vi "process.vi"(4 "error in":errorcluster, 6 "vars runtime":T1[](array[typedef])=[{"t wait"=5000, "t stim"=0, "t square"=0, "t rew"=0, "t onset"=0, "n stim"=0, "n hit"=0, "n miss"=0, "n catch"=0, "n reject"=0, "n false alarm"=0, "stim amp"=0.0, "stim idx"=0, "next temp"=0.0, "catch"=FALSE, "stimulus"=FALSE, "reward given"=FALSE, "lick"=FALSE, "next reward"=FALSE, "backlight"=FALSE, "square"=FALSE, "first run?"=TRUE, "run square?"=FALSE, "timeout"=FALSE, "free reward"=FALSE, "d stim"=0, "d square"=0, "n rew"=0}, {"t wait"=5000, "t stim"=0, "t square"=0, "t rew"=0, "t onset"=0, "n stim"=0, "n hit"=0, "n miss"=0, "n catch"=0, "n reject"=0, "n false alarm"=0, "stim amp"=0.0, "stim idx"=0, "next temp"=0.0, "catch"=FALSE, "stimulus"=FALSE, "reward given"=FALSE, "lick"=FALSE, "next reward"=FALSE, "backlight"=FALSE, "square"=FALSE, "first run?"=TRUE, "run square?"=FALSE, "timeout"=FALSE, "free reward"=FALSE, "d stim"=0, "d square"=0, "n rew"=0}, {"t wait"=5000, "t stim"=0, "t square"=0, "t rew"=0, "t onset"=0, "n stim"=0, "n hit"=0, "n miss"=0, "n catch"=0, "n reject"=0, "n false alarm"=0, "stim amp"=0.0, "stim idx"=0, "next temp"=0.0, "catch"=FALSE, "stimulus"=FALSE, "reward given"=FALSE, "lick"=FALSE, "next reward"=FALSE, "backlight"=FALSE, "square"=FALSE, "first run?"=TRUE, "run square?"=FALSE, "timeout"=FALSE, "free reward"=FALSE, "d stim"=0, "d square"=0, "n rew"=0}, {"t wait"=5000, "t stim"=0, "t square"=0, "t rew"=0, "t onset"=0, "n stim"=0, "n hit"=0, "n miss"=0, "n catch"=0, "n reject"=0, "n false alarm"=0, "stim amp"=0.0, "stim idx"=0, "next temp"=0.0, "catch"=FALSE, "stimulus"=FALSE, "reward given"=FALSE, "lick"=FALSE, "next reward"=FALSE, "backlight"=FALSE, "square"=FALSE, "first run?"=TRUE, "run square?"=FALSE, "timeout"=FALSE, "free reward"=FALSE, "d stim"=0, "d square"=0, "n rew"=0}], 7 "vars general":T2[](array[typedef])=[{"base directory"=path "C:/Users/training/Desktop/Data", "data directory"=path "C:/Users/training/Desktop/Data/animal001/session064", "active"=FALSE, "running"=FALSE, "pairing"=FALSE, "clean tubes"=FALSE, "animal ID"=1, "session ID"=64, "base temp"=32.0, "d wait min"=500, "d wait max"=1000, "d timeout"=5000, "d reward"=100, "n reward"=1, "idx stim"=0, "timeout win"=5000, "lick win"=[0, 100], "stim type"=[enum."pulse", enum."sine", enum."square"], "stim dur"=[500, 700, 600], "stim amp"=[10.0, 10.0, 10.0], "stim freq"=[50, 50, 50], "stim ramp"=[50, 1, 1], "stim catch"=[0, 0, 1], "square dur"=[50, 20, 10], "square delay"=[50, 20, 10], "square freq"=[50, 50, 50], "square dc"=[50, 20, 10], "stim shape"=array3x700[2100 elements], "square shape"=[[TRUE, TRUE, TRUE, TRUE, TRUE, TRUE, TRUE, TRUE, TRUE, TRUE, FALSE, FALSE, FALSE, FALSE, FALSE, FALSE, FALSE, FALSE, FALSE, FALSE, TRUE, TRUE, TRUE, TRUE, TRUE, TRUE, TRUE, TRUE, TRUE, TRUE, FALSE, FALSE, FALSE, FALSE, FALSE, FALSE, FALSE, FALSE, FALSE, FALSE, TRUE, TRUE, TRUE, TRUE, TRUE, TRUE, TRUE, TRUE, TRUE, TRUE], [TRUE, TRUE, TRUE, TRUE, FALSE, FALSE, FALSE, FALSE, FALSE, FALSE, FALSE, FALSE, FALSE, FALSE, FALSE, FALSE, FALSE, FALSE, FALSE, FALSE, FALSE, FALSE, FALSE, FALSE, FALSE, FALSE, FALSE, FALSE, FALSE, FALSE, FALSE, FALSE, FALSE, FALSE, FALSE, FALSE, FALSE, FALSE, FALSE, FALSE, FALSE, FALSE, FALSE, FALSE, FALSE, FALSE, FALSE, FALSE, FALSE, FALSE], [TRUE, TRUE, FALSE, FALSE, FALSE, FALSE, FALSE, FALSE, FALSE, FALSE, FALSE, FALSE, FALSE, FALSE, FALSE, FALSE, FALSE, FALSE, FALSE, FALSE, FALSE, FALSE, FALSE, FALSE, FALSE, FALSE, FALSE, FALSE, FALSE, FALSE, FALSE, FALSE, FALSE, FALSE, FALSE, FALSE, FALSE, FALSE, FALSE, FALSE, FALSE, FALSE, FALSE, FALSE, FALSE, FALSE, FALSE, FALSE, FALSE, FALSE]]}, {"base directory"=path "C:/Users/training/Desktop/Data", "data directory"=path "C:/Users/training/Desktop/Data/animal002/session122", "active"=FALSE, "running"=FALSE, "pairing"=FALSE, "clean tubes"=FALSE, "animal ID"=2, "session ID"=122, "base temp"=32.0, "d wait min"=500, "d wait max"=1000, "d timeout"=5000, "d reward"=100, "n reward"=1, "idx stim"=0, "timeout win"=5000, "lick win"=[0, 100], "stim type"=[enum."pulse", enum."sine", enum."square"], "stim dur"=[500, 700, 600], "stim amp"=[10.0, 10.0, 10.0], "stim freq"=[50, 50, 50], "stim ramp"=[50, 1, 1], "stim catch"=[0, 0, 1], "square dur"=[50, 20, 10], "square delay"=[50, 20, 10], "square freq"=[50, 50, 50], "square dc"=[50, 20, 10], "stim shape"=array3x700[2100 elements], "square shape"=[[TRUE, TRUE, TRUE, TRUE, TRUE, TRUE, TRUE, TRUE, TRUE, TRUE, FALSE, FALSE, FALSE, FALSE, FALSE, FALSE, FALSE, FALSE, FALSE, FALSE, TRUE, TRUE, TRUE, TRUE, TRUE, TRUE, TRUE, TRUE, TRUE, TRUE, FALSE, FALSE, FALSE, FALSE, FALSE, FALSE, FALSE, FALSE, FALSE, FALSE, TRUE, TRUE, TRUE, TRUE, TRUE, TRUE, TRUE, TRUE, TRUE, TRUE], [TRUE, TRUE, TRUE, TRUE, FALSE, FALSE, FALSE, FALSE, FALSE, FALSE, FALSE, FALSE, FALSE, FALSE, FALSE, FALSE, FALSE, FALSE, FALSE, FALSE, FALSE, FALSE, FALSE, FALSE, FALSE, FALSE, FALSE, FALSE, FALSE, FALSE, FALSE, FALSE, FALSE, FALSE, FALSE, FALSE, FALSE, FALSE, FALSE, FALSE, FALSE, FALSE, FALSE, FALSE, FALSE, FALSE, FALSE, FALSE, FALSE, FALSE], [TRUE, TRUE, FALSE, FALSE, FALSE, FALSE, FALSE, FALSE, FALSE, FALSE, FALSE, FALSE, FALSE, FALSE, FALSE, FALSE, FALSE, FALSE, FALSE, FALSE, FALSE, FALSE, FALSE, FALSE, FALSE, FALSE, FALSE, FALSE, FALSE, FALSE, FALSE, FALSE, FALSE, FALSE, FALSE, FALSE, FALSE, FALSE, FALSE, FALSE, FALSE, FALSE, FALSE, FALSE, FALSE, FALSE, FALSE, FALSE, FALSE, FALSE]]}, {"base directory"=path "C:/Users/training/Desktop/Data", "data directory"=path "C:/Users/training/Desktop/Data/animal003/session155", "active"=FALSE, "running"=FALSE, "pairing"=FALSE, "clean tubes"=FALSE, "animal ID"=3, "session ID"=155, "base temp"=32.0, "d wait min"=500, "d wait max"=1000, "d timeout"=5000, "d reward"=100, "n reward"=1, "idx stim"=0, "timeout win"=5000, "lick win"=[0, 100], "stim type"=[enum."pulse", enum."sine", enum."square"], "stim dur"=[500, 700, 600], "stim amp"=[10.0, 10.0, 10.0], "stim freq"=[50, 50, 50], "stim ramp"=[50, 1, 1], "stim catch"=[0, 0, 1], "square dur"=[50, 20, 10], "square delay"=[50, 20, 10], "square freq"=[50, 50, 50], "square dc"=[50, 20, 10], "stim shape"=array3x700[2100 elements], "square shape"=[[TRUE, TRUE, TRUE, TRUE, TRUE, TRUE, TRUE, TRUE, TRUE, TRUE, FALSE, FALSE, FALSE, FALSE, FALSE, FALSE, FALSE, FALSE, FALSE, FALSE, TRUE, TRUE, TRUE, TRUE, TRUE, TRUE, TRUE, TRUE, TRUE, TRUE, FALSE, FALSE, FALSE, FALSE, FALSE, FALSE, FALSE, FALSE, FALSE, FALSE, TRUE, TRUE, TRUE, TRUE, TRUE, TRUE, TRUE, TRUE, TRUE, TRUE], [TRUE, TRUE, TRUE, TRUE, FALSE, FALSE, FALSE, FALSE, FALSE, FALSE, FALSE, FALSE, FALSE, FALSE, FALSE, FALSE, FALSE, FALSE, FALSE, FALSE, FALSE, FALSE, FALSE, FALSE, FALSE, FALSE, FALSE, FALSE, FALSE, FALSE, FALSE, FALSE, FALSE, FALSE, FALSE, FALSE, FALSE, FALSE, FALSE, FALSE, FALSE, FALSE, FALSE, FALSE, FALSE, FALSE, FALSE, FALSE, FALSE, FALSE], [TRUE, TRUE, FALSE, FALSE, FALSE, FALSE, FALSE, FALSE, FALSE, FALSE, FALSE, FALSE, FALSE, FALSE, FALSE, FALSE, FALSE, FALSE, FALSE, FALSE, FALSE, FALSE, FALSE, FALSE, FALSE, FALSE, FALSE, FALSE, FALSE, FALSE, FALSE, FALSE, FALSE, FALSE, FALSE, FALSE, FALSE, FALSE, FALSE, FALSE, FALSE, FALSE, FALSE, FALSE, FALSE, FALSE, FALSE, FALSE, FALSE, FALSE]]}, {"base directory"=path "C:/Users/training/Desktop/Data", "data directory"=path "C:/Users/training/Desktop/Data/animal004/session061", "active"=FALSE, "running"=FALSE, "pairing"=FALSE, "clean tubes"=FALSE, "animal ID"=4, "session ID"=61, "base temp"=32.0, "d wait min"=500, "d wait max"=1000, "d timeout"=5000, "d reward"=100, "n reward"=1, "idx stim"=0, "timeout win"=5000, "lick win"=[0, 100], "stim type"=[enum."pulse", enum."sine", enum."square"], "stim dur"=[500, 700, 595], "stim amp"=[10.0, 10.0, 10.0], "stim freq"=[50, 50, 50], "stim ramp"=[50, 1, 1], "stim catch"=[0, 0, 1], "square dur"=[50, 20, 10], "square delay"=[50, 20, 10], "square freq"=[50, 50, 50], "square dc"=[50, 20, 10], "stim shape"=array3x700[2100 elements], "square shape"=[[TRUE, TRUE, TRUE, TRUE, TRUE, TRUE, TRUE, TRUE, TRUE, TRUE, FALSE, FALSE, FALSE, FALSE, FALSE, FALSE, FALSE, FALSE, FALSE, FALSE, TRUE, TRUE, TRUE, TRUE, TRUE, TRUE, TRUE, TRUE, TRUE, TRUE, FALSE, FALSE, FALSE, FALSE, FALSE, FALSE, FALSE, FALSE, FALSE, FALSE, TRUE, TRUE, TRUE, TRUE, TRUE, TRUE, TRUE, TRUE, TRUE, TRUE], [TRUE, TRUE, TRUE, TRUE, FALSE, FALSE, FALSE, FALSE, FALSE, FALSE, FALSE, FALSE, FALSE, FALSE, FALSE, FALSE, FALSE, FALSE, FALSE, FALSE, FALSE, FALSE, FALSE, FALSE, FALSE, FALSE, FALSE, FALSE, FALSE, FALSE, FALSE, FALSE, FALSE, FALSE, FALSE, FALSE, FALSE, FALSE, FALSE, FALSE, FALSE, FALSE, FALSE, FALSE, FALSE, FALSE, FALSE, FALSE, FALSE, FALSE], [TRUE, TRUE, FALSE, FALSE, FALSE, FALSE, FALSE, FALSE, FALSE, FALSE, FALSE, FALSE, FALSE, FALSE, FALSE, FALSE, FALSE, FALSE, FALSE, FALSE, FALSE, FALSE, FALSE, FALSE, FALSE, FALSE, FALSE, FALSE, FALSE, FALSE, FALSE, FALSE, FALSE, FALSE, FALSE, FALSE, FALSE, FALSE, FALSE, FALSE, FALSE, FALSE, FALSE, FALSE, FALSE, FALSE, FALSE, FALSE, FALSE, FALSE]]}] {"stim ramp" min=1}) -> (0 "error out":errorcluster, 2 "vars runtime":T1[](array[typedef])=[{"t wait"=5000, "t stim"=0, "t square"=0, "t rew"=0, "t onset"=0, "n stim"=0, "n hit"=0, "n miss"=0, "n catch"=0, "n reject"=0, "n false alarm"=0, "stim amp"=0.0, "stim idx"=0, "next temp"=32.0, "catch"=FALSE, "stimulus"=FALSE, "reward given"=FALSE, "lick"=FALSE, "next reward"=FALSE, "backlight"=FALSE, "square"=FALSE, "first run?"=TRUE, "run square?"=FALSE, "timeout"=FALSE, "free reward"=FALSE, "d stim"=0, "d square"=0, "n rew"=0}, {"t wait"=5000, "t stim"=0, "t square"=0, "t rew"=0, "t onset"=0, "n stim"=0, "n hit"=0, "n miss"=0, "n catch"=0, "n reject"=0, "n false alarm"=0, "stim amp"=0.0, "stim idx"=0, "next temp"=32.0, "catch"=FALSE, "stimulus"=FALSE, "reward given"=FALSE, "lick"=FALSE, "next reward"=FALSE, "backlight"=FALSE, "square"=FALSE, "first run?"=TRUE, "run square?"=FALSE, "timeout"=FALSE, "free reward"=FALSE, "d stim"=0, "d square"=0, "n rew"=0}, {"t wait"=5000, "t stim"=0, "t square"=0, "t rew"=0, "t onset"=0, "n stim"=0, "n hit"=0, "n miss"=0, "n catch"=0, "n reject"=0, "n false alarm"=0, "stim amp"=0.0, "stim idx"=0, "next temp"=32.0, "catch"=FALSE, "stimulus"=FALSE, "reward given"=FALSE, "lick"=FALSE, "next reward"=FALSE, "backlight"=FALSE, "square"=FALSE, "first run?"=TRUE, "run square?"=FALSE, "timeout"=FALSE, "free reward"=FALSE, "d stim"=0, "d square"=0, "n rew"=0}, {"t wait"=5000, "t stim"=0, "t square"=0, "t rew"=0, "t onset"=0, "n stim"=0, "n hit"=0, "n miss"=0, "n catch"=0, "n reject"=0, "n false alarm"=0, "stim amp"=0.0, "stim idx"=0, "next temp"=32.0, "catch"=FALSE, "stimulus"=FALSE, "reward given"=FALSE, "lick"=FALSE, "next reward"=FALSE, "backlight"=FALSE, "square"=FALSE, "first run?"=TRUE, "run square?"=FALSE, "timeout"=FALSE, "free reward"=FALSE, "d stim"=0, "d square"=0, "n rew"=0}])   [LabVIEW 2016]
uses:
  Type Definitions/vars_settings.ctl
  Type Definitions/stim_type.ctl
  Type Definitions/vars_runtime.ctl
  Type Definitions/states.ctl
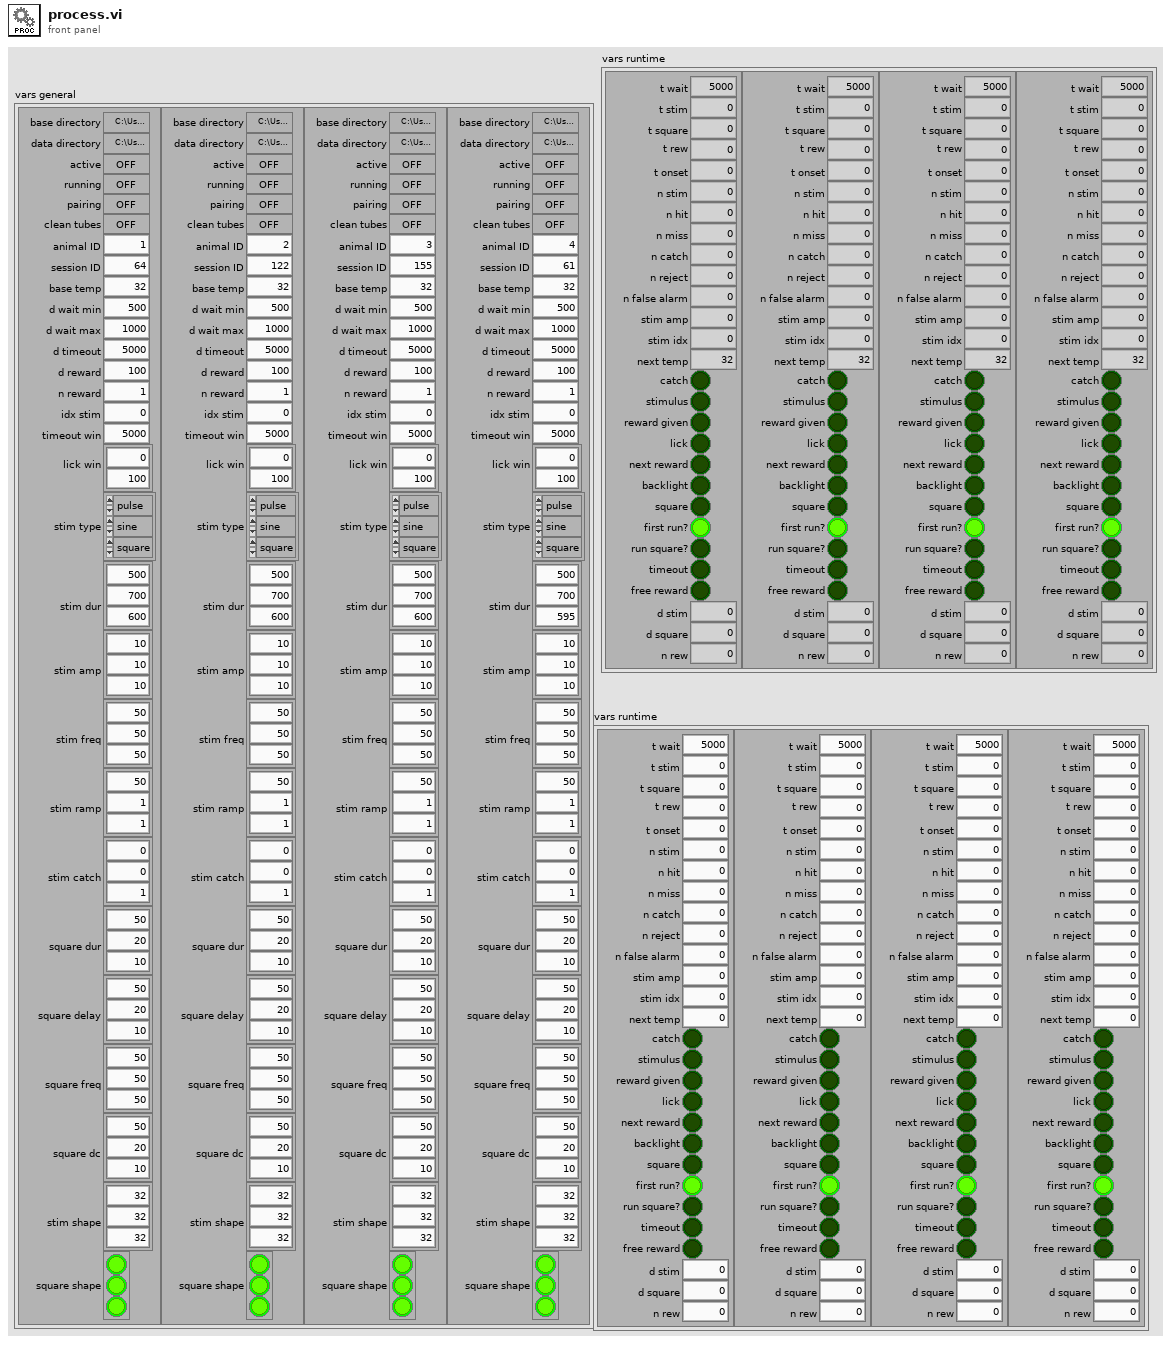
[diagram p1: front panel]
types:
  T1 = typedef "vars_runtime.ctl" = cluster{"t wait":u16, "t stim":u16, "t square":u16, "t rew":u16, "t onset":u32, "n stim":u16, "n hit":u16, "n miss":u16, "n catch":u16, "n reject":u16, "n false alarm":u16, "stim amp":sgl, "stim idx":i32, "next temp":sgl, "catch":bool, "stimulus":bool, "reward given":bool, "lick":bool, "next reward":bool, "backlight":bool, "square":bool, "first run?":bool, "run square?":bool, "timeout":bool, "free reward":bool, "d stim":u16, "d square":u16, "n rew":u16}
  T2 = typedef "vars_settings.ctl" = cluster{"base directory":path, "data directory":path, "active":bool, "running":bool, "pairing":bool, "clean tubes":bool, "animal ID":u16, "session ID":u16, "base temp":dbl, "d wait min":u16, "d wait max":u16, "d timeout":u16, "d reward":u16, "n reward":u16, "idx stim":u16, "timeout win":u16, "lick win":i32[], "stim type":T3[], "stim dur":u16[], "stim amp":dbl[], "stim freq":u16[], "stim ramp":u16[], "stim catch":u8[], "square dur":u16[], "square delay":i16[], "square freq":u8[], "square dc":u8[], "stim shape":dbl[][], "square shape":bool[][]}
  T3 = typedef "stim_type.ctl" = enum16{"pulse", "vibration", "square", "sine"}
  T4 = typedef "states.ctl" = enum16{"initialize", "lick", "lick reward", "lick timeout", "wait", "initialize stimulus", "stimulus", "backlight", "inactive", "shutdown", "squarewave"}
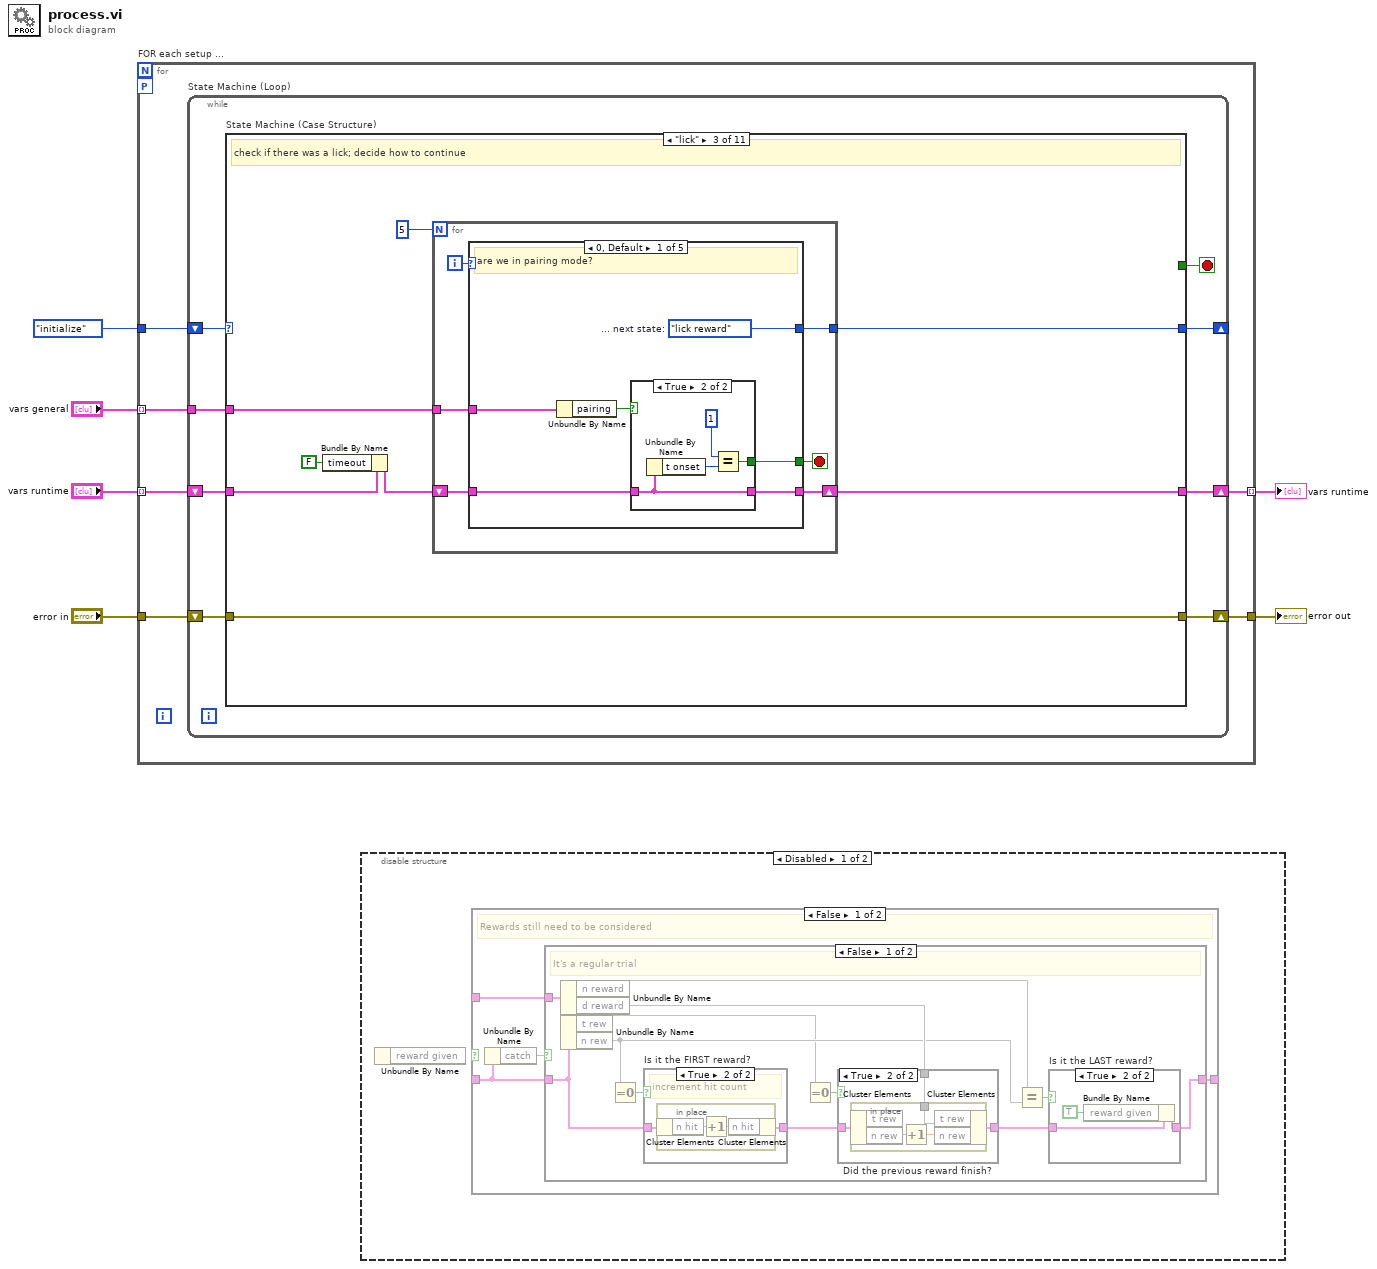
[diagram p0: block diagram]
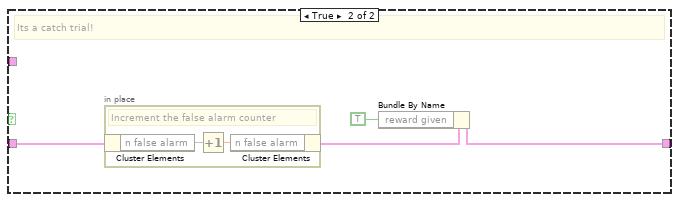
[diagram p5: hidden frame]
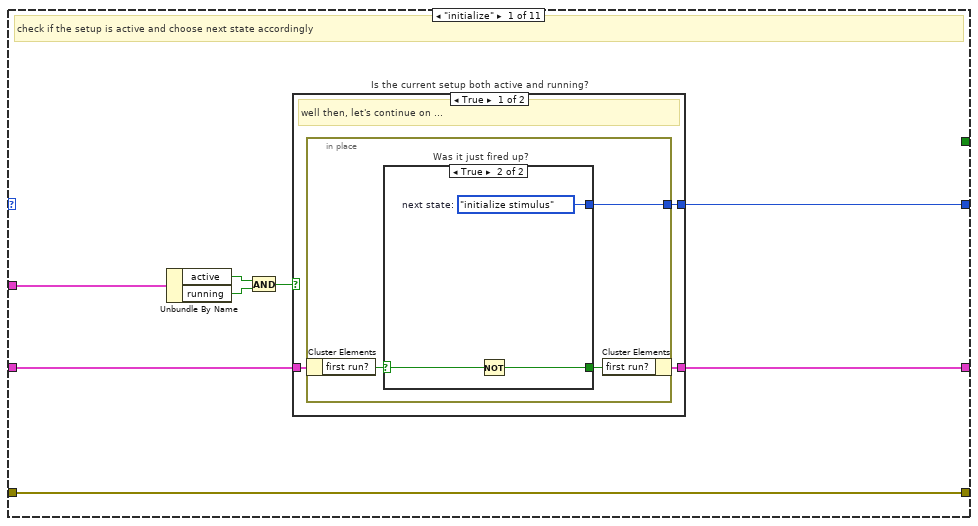
[diagram p8: hidden frame]
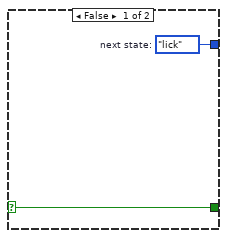
[diagram p9: hidden frame]
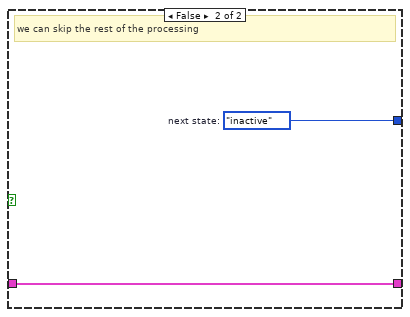
[diagram p10: hidden frame]
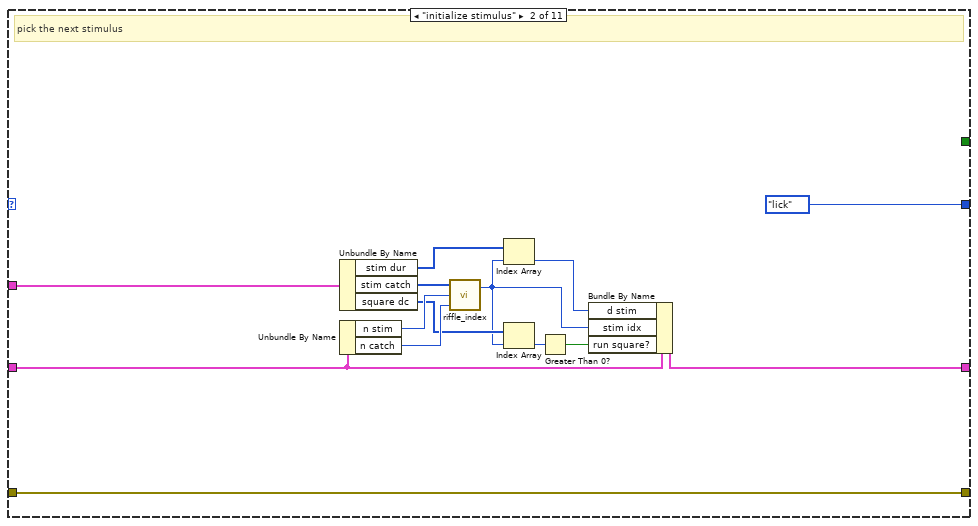
[diagram p11: hidden frame]
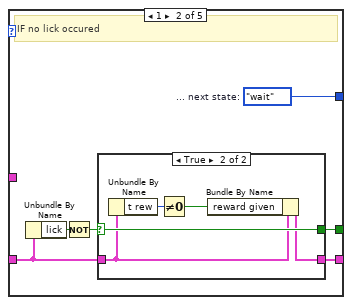
[diagram p13: hidden frame]
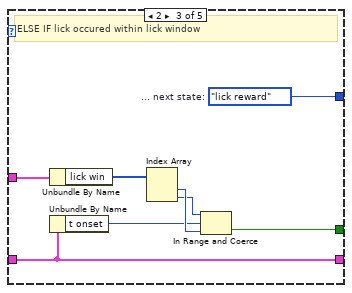
[diagram p15: hidden frame]
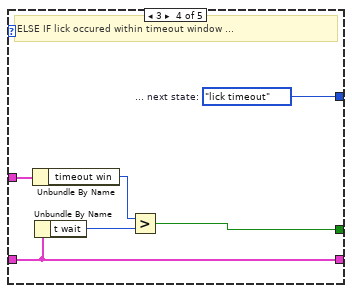
[diagram p16: hidden frame]
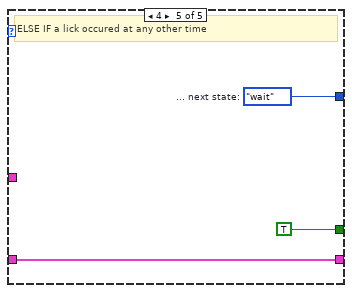
[diagram p17: hidden frame]
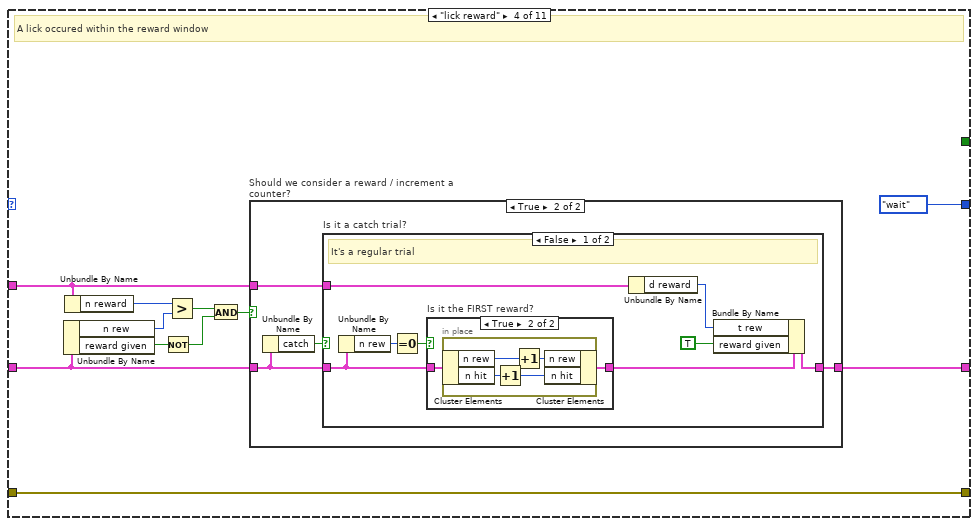
[diagram p18: hidden frame]
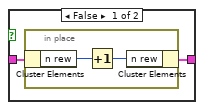
[diagram p20: hidden frame]
diagram:
  n1 = for "FOR each setup ..." {
    tunnel: "error in" -> [w12]
    tunnel: [w11] -> w6
    tunnel: "vars runtime" -> [w7] mode=indexing
    tunnel: [w9] -> w3 mode=indexing
    tunnel: states."initialize" ("initial state") -> [w10]
    tunnel: "vars general" -> [w8] mode=indexing
    workers-P: _ -> [_]
    n2 = while "State Machine (Loop)" {
      shift-right: [w20] -> w11
      shift-left: w12 -> [w18]
      shift-right: [w16] -> _
      shift-left: w10 -> [w17]
      shift-right: [w13] -> w9
      shift-left: w7 -> [w14]
      tunnel: w8 -> [w15]
      stop <- w19 stop-if-true
      n3 = case "State Machine (Case Structure)" shown="\"lick\"" w17 {
        tunnel: [w28 w55 w60 w112 w159 w165 w228 w266 w316 w332 w348] -> w20
        tunnel: w18 -> [w28 w55 w60 w112 w159 w165 w228 w266 w316 w332 w348]
        tunnel: w14 -> [w22 w50 w58 w121 w160 w171 w229 w264 w309 w328 w343]
        tunnel: [_ _ _ _ _ _ _ _ _ _ TRUE] -> w19
        tunnel: [w27 states."lick" ("next state:") w59 states."wait" ("next state:") states."wait" ("next state:") states."squarewave" ("next state:") w225 states."stimulus" ("next state:") states."shutdown" ("next state:") w330 w347] -> w16
        tunnel: w15 -> [w26 w48 w61 w119 w157 w172 w223 w259 w308 w333 w345]
        tunnel: [w21 w49 w62 w120 w155 w167 w218 w261 w314 w331 w344] -> w13
        frame "initialize" {
          # "check if the setup is active and choose next state accordingly"
          n4 = Unbundle By Name(w26) -> ("active"=w24:bool, "running"=w23:bool)
          n5 = And(x=w24, y=w23) -> (x .and. y?=w25:bool)
          n6 = case "Is the current setup both active and running?" shown="True" w25 {
            tunnel: [w31 w41] -> w27
            tunnel: w22 -> [w30 w40]
            tunnel: [w29 w40] -> w21
            frame True {
              # "well then, let's continue on ..."
              n7 = in-place {
                in-place-border: [w34] -> w31
                n8 = in-place-cluster #1(w30) -> ("first run?"=w33:bool)
                n9 = case "Was it just fired up?" shown="True" w33 {
                  selector: w33 -> [w35 w38]
                  tunnel: [w36 w39] -> w34
                  tunnel: [w35 w37] -> w32
                  frame False {
                    w36 = states."lick"  # next state:
                  }
                  frame True {
                    w39 = states."initialize stimulus"  # next state:
                    n10 = Not(x=w38) -> (.not. x?=w37:bool)
                  }
                }
                n11 = in-place-cluster #1("first run?"=w32) -> (w29:T1)
              }
            }
            frame False {
              w41 = states."inactive"  # next state:
              # "we can skip the rest of the processing"
            }
          }
        }
        frame "initialize stimulus" {
          # "pick the next stimulus"
          n12 = Unbundle By Name(w48) -> ("stim dur"=w53:u16[], "stim catch"=w54:u8[], "square dc"=w45:u8[])
          n13 = Unbundle By Name(w50) -> ("n stim"=w52:u16, "n catch"=w51:u16)
          n14 = call "riffle_index.vi"("n catch"=w51, "n stim"=w52, "stim array in"=w54) -> ("riffled index"=w42:i32)  [unwired: 1 out]
          n15 = Index Array(array=w53, index=w42) -> (element=w46:u16)
          n16 = Index Array(array=w45, index=w42) -> (element=w44:u8)
          n17 = Greater Than 0?(x=w44) -> (x > 0?=w43:bool)
          n18 = Bundle By Name(cluster=w50, "d stim"=w46, "stim idx"=w42, "run square?"=w43) -> (w49:T1)
        }
        frame "lick" {
          # "check if there was a lick; decide how to continue"
          n19 = Bundle By Name(cluster=w58, "timeout"=FALSE) -> (w57:T1)
          n20 = for {
            N: 5 -> [_]
            tunnel: [w66] -> w59
            shift-right: [w65] -> w62
            shift-left: w57 -> [w67]
            tunnel: w61 -> [w64]
            i -> [w69]
            stop <- w68 stop-if-true
            # "If-then-else-if ..."
            n21 = case shown="0, Default" w69 {
              tunnel: [w72 w84 w95 w105 TRUE] -> w68
              tunnel: w67 -> [w73 w83 w97 w107 w111]
              tunnel: [w71 w87 w102 w108 w109] -> w66
              tunnel: [w70 w82 w97 w107 w111] -> w65
              tunnel: w64 -> [w75 _ w98 w106 _]
              frame 0, Default {
                w71 = states."lick reward"  # ... next state:
                # "are we in pairing mode?"
                n22 = Unbundle By Name(w75) -> ("pairing"=w74:bool)
                n23 = case shown="True" w74 {
                  selector: w74 -> [w77 _]
                  tunnel: w73 -> [w76 w81]
                  tunnel: [w77 w78] -> w72
                  tunnel: [w76 w81] -> w70
                  frame False {
                  }
                  frame True {
                    n24 = Unbundle By Name(w81) -> ("t onset"=w80:u32)
                    n25 = Equal?(x=u32 1, y=w80) -> (x = y?=w78:bool)
                  }
                }
              }
              frame 1 {
                w87 = states."wait"  # ... next state:
                # "IF no lick occured"
                n26 = Unbundle By Name(w83) -> ("lick"=w86:bool)
                n27 = Not(x=w86) -> (.not. x?=w85:bool)
                n28 = case shown="True" w85 {
                  selector: w85 -> [w88 w94]
                  tunnel: [w88 w94] -> w84
                  tunnel: w83 -> [w89 w92]
                  tunnel: [w89 w91] -> w82
                  frame False {
                  }
                  frame True {
                    n29 = Unbundle By Name(w92) -> ("t rew"=w93:u16)
                    n30 = Not Equal To 0?(x=w93) -> (x != 0?=w90:bool)
                    n31 = Bundle By Name(cluster=w92, "reward given"=w90) -> (w91:T1)
                  }
                }
              }
              frame 2 {
                w102 = states."lick reward"  # ... next state:
                # "ELSE IF lick occured within lick window"
                n32 = Unbundle By Name(w98) -> ("lick win"=w101:i32[])
                n33 = Unbundle By Name(w97) -> ("t onset"=w96:u32)
                n34 = Index Array(array=w101) -> (element #1=w100:i32, element #2=w99:i32)  [unwired: 2 in]
                n35 = In Range and Coerce(upper limit=w99, x=w96, lower limit=w100) -> (In Range?=w95:bool)  [unwired: 1 out]
              }
              frame 3 {
                w108 = states."lick timeout"  # ... next state:
                # "ELSE IF lick occured within timeout window ..."
                n36 = Unbundle By Name(w106) -> ("timeout win"=w103:u16)
                n37 = Unbundle By Name(w107) -> ("t wait"=w104:u16)
                n38 = Greater?(x=w103, y=w104) -> (0:w105:bool)
              }
              frame 4 {
                w109 = states."wait"  # ... next state:
                # "ELSE IF a lick occured at any other time"
              }
            }
          }
        }
        frame "lick reward" {
          # "A lick occured within the reward window"
          n39 = Unbundle By Name(w121) -> ("n rew"=w117:u16, "reward given"=w115:bool)
          n40 = Unbundle By Name(w119) -> ("n reward"=w118:u16)
          n41 = Not(x=w115) -> (.not. x?=w116:bool)
          n42 = Greater?(x=w118, y=w117) -> (0:w114:bool)
          n43 = And(x=w114, y=w116) -> (x .and. y?=w113:bool)
          n44 = case "Should we consider a reward / increment a counter?" shown="True" w113 {
            tunnel: w121 -> [w123 w127]
            tunnel: w119 -> [_ w126]
            tunnel: [w123 w125] -> w120
            frame False {
            }
            frame True {
              n45 = Unbundle By Name(w127) -> ("catch"=w124:bool)
              n46 = case "Is it a catch trial?" shown="False" w124 {
                tunnel: w127 -> [w135 w151]
                tunnel: w126 -> [w134 w147]
                tunnel: [w129 w149] -> w125
                frame False {
                  # "It's a regular trial"
                  n47 = Unbundle By Name(w135) -> ("n rew"=w132:u16)
                  n48 = Equal To 0?(x=w132) -> (x = 0?=w133:bool)
                  n49 = case "Is it the FIRST reward?" shown="True" w133 {
                    tunnel: w135 -> [w137 w141]
                    tunnel: [w136 w140] -> w130
                    frame False {
                      # "increment hit count"
                      n50 = in-place {
                        # "Increment hit counter"
                        n51 = in-place-cluster #2(w137) -> ("n rew"=w139:u16)
                        n52 = Increment(x=w139) -> (x+1=w138:u16)
                        n53 = in-place-cluster #2("n rew"=w138) -> (w136:T1)
                      }
                    }
                    frame True {
                      # "increment hit count"
                      n54 = in-place {
                        # "Increment hit counter"
                        n55 = in-place-cluster #3(w141) -> ("n rew"=w143:u16, "n hit"=w144:u16)
                        n56 = Increment(x=w144) -> (x+1=w145:u16)
                        n57 = Increment(x=w143) -> (x+1=w142:u16)
                        n58 = in-place-cluster #3("n rew"=w142, "n hit"=w145) -> (w140:T1)
                      }
                    }
                  }
                  n59 = Unbundle By Name(w134) -> ("d reward"=w128:u16)
                  n60 = Bundle By Name(cluster=w130, "t rew"=w128, "reward given"=TRUE) -> (w129:T1)
                }
                frame True {
                  # "Its a catch trial!"
                  n61 = in-place {
                    # "Increment the false alarm counter"
                    n62 = in-place-cluster #4(w151) -> ("n false alarm"=w153:u16)
                    n63 = Increment(x=w153) -> (x+1=w152:u16)
                    n64 = in-place-cluster #4("n false alarm"=w152) -> (w148:T1)
                  }
                  n65 = Unbundle By Name(w147) -> ("n reward"=w146:u16)
                  n66 = Bundle By Name(cluster=w148, "n rew"=w146, "reward given"=TRUE) -> (w149:T1)
                }
              }
            }
          }
        }
        frame "lick timeout" {
          # "add timeout period to the wait counter"
          n67 = in-place {
            in-place-border: w157 -> [w162]
            # "add timeout to wait counter"
            n68 = in-place-cluster #5(w160) -> ("t wait"=w164:u16)
            n69 = Unbundle By Name(w162) -> ("d timeout"=w161:u16)
            n70 = Add(x=w161, y=w164) -> (x+y=w163:u16)
            n71 = in-place-cluster #5("t wait"=w163) -> (w156:T1)
          }
          n72 = Bundle By Name(cluster=w156, "timeout"=TRUE) -> (w155:T1)
        }
        frame "wait" {
          n73 = Unbundle By Name(w171) -> ("t wait"=w170:u16)
          n74 = case shown="0" w170 {
            selector: w170 -> [w189 _]
            tunnel: [w188 w192] -> w169
            tunnel: w172 -> [_ w207]
            tunnel: w171 -> [w187 w200]
            tunnel: [w187 w194] -> w168
            frame Default {
              # "decrement wait counter"
              n75 = Decrement(x=w189) -> (x-1=w188:u16)
            }
            frame 0 {
              # "initialize stimulus"
              n76 = Unbundle By Name(w207) -> ("d wait max"=w205:u16, "d wait min"=w201:u16, "stim catch"=w208:u8[])
              n77 = Unbundle By Name(w200) -> ("d stim"=w199:u16, "stim idx"=w198:i32)
              n78 = Subtract(x=w205, y=w201) -> (x-y=w204:u16)
              n79 = Index Array(array=w208, index=w198) -> (element=w197:u8)
              n80 = Bundle By Name(cluster=w200, "t stim"=w199, "stimulus"=TRUE, "t onset"=u32 0, "n rew"=u16 0 ("t since onset")) -> (w195:T1)
              n81 = Random Number (0-1)() -> (number: 0 to 1=w206:dbl)
              n82 = Multiply(x=w206, y=w204) -> (x*y=w203:dbl)
              n83 = Greater Than 0?(x=w197) -> (x > 0?=w196:bool)
              n84 = To Unsigned Word Integer(number=w203) -> (unsigned 16bit integer=w202:u16)
              n85 = Compound Arithmetic op=ADD(w202, w201, w199) -> (w192:u16)
              n86 = case shown="True" w196 {
                tunnel: w195 -> [w210 w214]
                tunnel: [w209 w213] -> w194
                frame False {
                  n87 = in-place {
                    n88 = in-place-cluster #6(w210) -> ("n stim"=w212:u16)
                    n89 = Increment(x=w212) -> (x+1=w211:u16)
                    n90 = in-place-cluster #6("n stim"=w211) -> (w209:T1)
                  }
                }
                frame True {
                  n91 = in-place {
                    n92 = in-place-cluster #7(w214) -> ("n catch"=w217:u16)  [unwired: 1 out]
                    n93 = Increment(x=w217) -> (x+1=w216:u16)
                    n94 = in-place-cluster #7("catch"=TRUE, "n catch"=w216) -> (w213:T1)
                  }
                }
              }
            }
          }
          n95 = Bundle By Name(cluster=w168, "t wait"=w169) -> (w166:T1)
          n96 = in-place {
            n97 = in-place-cluster #8(w166) -> ("free reward"=w175:bool, "t rew"=w179:u16, "t onset"=w177:u32)  [unwired: 1 out]
            n98 = case shown="0" w179 {
              selector: w179 -> [w182 w185]
              tunnel: [w182 w186] -> w180
              tunnel: [w181 TRUE] -> w178
              tunnel: w175 -> [_ w183]
              tunnel: [w181 w183] -> w174
              frame 0 {
                w181 = FALSE
                # "do nothing"
              }
              frame Default {
                # "decrement reward counter"
                n99 = Decrement(x=w185) -> (x-1=w186:u16)
              }
            }
            n100 = Increment(x=w177) -> (x+1=w176:u32)
            n101 = in-place-cluster #8("free reward"=w174, "next reward"=w178, "t rew"=w180, "t onset"=w176) -> (w167:T1)
          }
        }
        frame "stimulus" {
          n102 = Unbundle By Name(w229) -> ("t stim"=w227:u16)
          n103 = Greater Than 0?(x=w227) -> (x > 0?=w226:bool)
          n104 = case shown="True" w226 {
            tunnel: w229 -> [w239 w243]
            tunnel: [w238 w244] -> w219
            tunnel: w223 -> [w237 w245]
            tunnel: [w235 w240] -> w225
            frame False {
              w235 = states."backlight"  # next state
              # "set base conditions"
              n105 = Unbundle By Name(w237) -> ("base temp"=w236:dbl)
              n106 = Bundle By Name(cluster=w239, "next temp"=w236, "stimulus"=FALSE) -> (w238:T1)
            }
            frame True {
              # "play stimulus"
              n107 = Unbundle By Name(w245) -> ("stim shape"=w251:dbl[][])
              n108 = Unbundle By Name(w243) -> ("stim idx"=w250:i32, "d stim"=w248:u16, "t stim"=w247:u16)
              n109 = Subtract(x=w248, y=w247) -> (x-y=w246:u16)
              n110 = Index Array(array=w251, index (row)=w250, index (col)=w246) -> (element=w249:dbl)
              n111 = Decrement(x=w247) -> (x-1=w242:u16)
              n112 = Equal To 0?(x=w242) -> (x = 0?=w241:bool)
              n113 = Bundle By Name(cluster=w243, "next temp"=w249, "t stim"=w242) -> (w244:T1)
              n114 = case "End of current stimulus?" shown="True" w241 {
                tunnel: [w252 w253] -> w240
                frame False {
                  w252 = states."backlight"  # next state
                }
                frame True {
                  w253 = states."initialize stimulus"  # next state
                }
              }
            }
          }
          n115 = Unbundle By Name(w223) -> ("lick win"=w222:i32[])
          n116 = Unbundle By Name(w219) -> ("t onset"=w224:u32)
          n117 = Index Array(array=w222) -> (element #2=w221:i32)  [unwired: 2 in, 1 out]
          n118 = Greater?(x=w224, y=w221) -> (0:w220:bool)
          n119 = case shown="False" w220 {
            tunnel: w219 -> [w230 w233]
            tunnel: [w230 w232] -> w218
            frame False {
            }
            frame True {
              n120 = Bundle By Name(cluster=w233, "catch"=FALSE) -> (w232:T1)
            }
          }
        }
        frame "squarewave" {
          n121 = Unbundle By Name(w264) -> ("t square"=w257:u16, "run square?"=w255:bool)
          n122 = Equal To 0?(x=w257) -> (x = 0?=w254:bool)
          n123 = And(x=w254, y=w255) -> (x .and. y?=w256:bool)
          n124 = case shown="True" w256 {
            tunnel: w264 -> [w281 w284]
            tunnel: [w281 w288] -> w262
            tunnel: w259 -> [w280 w282]
            tunnel: [w280 w282] -> w258
            frame False {
            }
            frame True {
              n125 = Unbundle By Name(w282) -> ("square dur"=w286:u16[], "square delay"=w285:i16[])
              n126 = Unbundle By Name(w284) -> ("stim idx"=w283:i32)
              n127 = Index Array(array=w285, index=w283) -> (element=w290:i16)
              n128 = Less Or Equal To 0?(x=w290) -> (x <= 0?=w291:bool)
              n129 = case shown="True" w291 {
                tunnel: w290 -> [w298 w304]
                tunnel: w284 -> [w299 w305]
                tunnel: [w300 w306] -> w287
                tunnel: [w299 w305] -> w289
                frame False {
                  n130 = Unbundle By Name(w299) -> ("t onset"=w301:u32)
                  n131 = Equal?(x=w298, y=w301) -> (x = y?=w300:bool)
                }
                frame True {
                  n132 = Negate(x=w304) -> (-x=w303:i16)
                  n133 = Unbundle By Name(w305) -> ("t wait"=w307:u16)
                  n134 = To Unsigned Word Integer(number=w303) -> (unsigned 16bit integer=w302:u16)
                  n135 = Equal?(x=w302, y=w307) -> (x = y?=w306:bool)
                }
              }
              n136 = case shown="True" w287 {
                tunnel: w289 -> [w292 w297]
                tunnel: [w292 w296] -> w288
                tunnel: w286 -> [_ w295]
                tunnel: w283 -> [_ w293]
                frame False {
                }
                frame True {
                  n137 = Index Array(array=w295, index=w293) -> (element=w294:u16)
                  n138 = Bundle By Name(cluster=w297, "d square"=w294, "t square"=w294) -> (w296:T1)
                }
              }
            }
          }
          n139 = Unbundle By Name(w262) -> ("t square"=w263:u16)
          n140 = Greater Than 0?(x=w263) -> (x > 0?=w260:bool)
          n141 = case shown="True" w260 {
            tunnel: w262 -> [w269 w274]
            tunnel: [w268 w273] -> w261
            tunnel: w258 -> [_ w279]
            frame False {
              n142 = Bundle By Name(cluster=w269, "square"=FALSE) -> (w268:T1)
            }
            frame True {
              n143 = Unbundle By Name(w279) -> ("square shape"=w278:bool[][])
              n144 = Unbundle By Name(w274) -> ("stim idx"=w270:i32, "d square"=w277:u16, "t square"=w272:u16)
              n145 = Subtract(x=w277, y=w272) -> (x-y=w276:u16)
              n146 = Decrement(x=w272) -> (x-1=w271:u16)
              n147 = Index Array(array=w278, index (row)=w270, index (col)=w276) -> (element=w275:bool)
              n148 = Bundle By Name(cluster=w274, "square"=w275, "t square"=w271) -> (w273:T1)
            }
          }
        }
        frame "backlight" {
          w313 = u32 100  # period
          # "a randomized digital output with a given period, switching states with a defined probability"
          n149 = Tick Count (ms)() -> (millisecond timer value=w310:u32)
          n150 = Quotient & Remainder(x=w310, y=w313) -> (x-y*floor(x/y)=w312:u32)  [unwired: 1 out]
          n151 = Equal To 0?(x=w312) -> (x = 0?=w311:bool)
          n152 = case shown="True" w311 {
            tunnel: w309 -> [w317 w322]
            tunnel: [w317 w321] -> w314
            tunnel: w308 -> [_ _]
            frame False {
            }
            frame True {
              w318 = 0.25  # probability
              n153 = Random Number (0-1)() -> (number: 0 to 1=w320:dbl)
              n154 = Less Or Equal?(x=w320, y=w318) -> (x <= y?=w319:bool)
              n155 = case shown="True" w319 {
                tunnel: w322 -> [w323 w325]
                tunnel: [w323 w324] -> w321
                frame False {
                }
                frame True {
                  n156 = in-place {
                    n157 = in-place-cluster #9(w325) -> ("backlight"=w327:bool)
                    n158 = Not(x=w327) -> (.not. x?=w326:bool)
                    n159 = in-place-cluster #9("backlight"=w326) -> (w324:T1)
                  }
                }
              }
            }
          }
        }
        frame "inactive" {
          w330 = states."shutdown"  # next state:
          n160 = Unbundle By Name(w328) -> ("first run?"=w329:bool)
          n161 = case shown="False" w329 {
            tunnel: w333 -> [w340 _]
            tunnel: [w339 w341] -> w331
            tunnel: w328 -> [_ w341]
            frame False {
              n162 = Unbundle By Name(w340) -> ("base temp"=w337:dbl, "d wait max"=w336:u16)
              n163 = Bundle By Name(cluster=T1 {"t wait"=0, "t stim"=0, "t square"=0, "t rew"=0, "t onset"=0, "n stim"=0, "n hit"=0, "n miss"=0, "n catch"=0, "n reject"=0, "n false alarm"=0, "stim amp"=0.0, "stim idx"=0, "next temp"=0.0, "catch"=FALSE, "stimulus"=FALSE, "reward given"=FALSE, "lick"=FALSE, "next reward"=FALSE, "backlight"=FALSE, "square"=FALSE, "first run?"=FALSE, "run square?"=FALSE, "timeout"=FALSE, "free reward"=FALSE, "d stim"=0, "d square"=0, "n rew"=0} ("Cluster"), "next temp"=w337, "t wait"=w336, "t onset"=u16 10000 ("t since onset"), "first run?"=TRUE) -> (w339:T1)
            }
            frame True {
            }
          }
        }
        frame "shutdown" {
          w347 = states."initialize"  # next state:
          # "perform final tasks and exit state machine"
          n164 = Unbundle By Name(w345) -> ("clean tubes"=w342:bool)
          n165 = in-place {
            in-place-border: w342 -> [w349]
            n166 = in-place-cluster #10(w343) -> ("next reward"=w351:bool)
            n167 = Or(x=w349, y=w351) -> (x .or. y?=w350:bool)
            n168 = in-place-cluster #10("next reward"=w350) -> (w344:T1)
          }
        }
      }
    }
  }
  "error out" <- w6
  "vars runtime" <- w3
  n169 = disable-structure shown="Disabled" {
    frame Disabled {
      n170 = Unbundle By Name() -> ()  [unwired: 1 in, 1 out]
      n171 = case shown="False" {
        selector: _ -> [_ _]
        tunnel: _ -> [w354 w390]
        tunnel: _ -> [w353 _]
        tunnel: [w352 w390] -> _
        frame False {
          # "Rewards still need to be considered"
          n172 = Unbundle By Name(w354) -> ("catch"=w355)
          n173 = case shown="False" w355 {
            tunnel: w354 -> [w367 w387]
            tunnel: w353 -> [w366 _]
            tunnel: [w364 w385] -> w352
            frame False {
              # "It's a regular trial"
              n174 = Unbundle By Name(w366) -> ("n reward"=w365, "d reward"=w359)
              n175 = Unbundle By Name(w367) -> ("t rew"=w356, "n rew"=w358)
              n176 = Equal To 0?(x=w358) -> (x = 0?=w360:bool)
              n177 = case "Is it the FIRST reward?" shown="True" w360 {
                tunnel: w367 -> [w379 w381]
                tunnel: [w379 w380] -> w362
                frame False {
                  # "do nothing"
                }
                frame True {
                  # "increment hit count"
                  n178 = in-place {
                    # "Increment hit counter"
                    n179 = in-place-cluster #11(w381) -> ("n hit"=w382)
                    n180 = Increment(x=w382) -> (x+1=w383:dbl)
                    n181 = in-place-cluster #11("n hit"=w383) -> (w380:cluster{})
                  }
                }
              }
              n182 = Equal To 0?(x=w356) -> (x = 0?=w357:bool)
              n183 = case "Did the previous reward finish?" shown="True" w357 {
                tunnel: w362 -> [w368 w371]
                tunnel: [w368 w370] -> w361
                tunnel: w359 -> [_ w369]
                frame False {
                }
                frame True {
                  n184 = in-place {
                    in-place-border: w369 -> [w372]
                    # "Increment hit counter"
                    n185 = in-place-cluster #12(w371) -> ("n rew"=w374)  [unwired: 1 out]
                    n186 = Increment(x=w374) -> (x+1=w373:dbl)
                    n187 = in-place-cluster #12("t rew"=w372, "n rew"=w373) -> (w370:cluster{})
                  }
                }
              }
              n188 = Equal?(x=w365, y=w358) -> (x = y?=w363:bool)
              n189 = case "Is it the LAST reward?" shown="True" w363 {
                tunnel: w361 -> [w375 w378]
                tunnel: [w375 w377] -> w364
                frame False {
                }
                frame True {
                  n190 = Bundle By Name(cluster=w378, "reward given"=TRUE ("reward done")) -> (w377:cluster{})
                }
              }
            }
            frame True {
              # "Its a catch trial!"
              n191 = in-place {
                # "Increment the false alarm counter"
                n192 = in-place-cluster #13(w387) -> ("n false alarm"=w389)
                n193 = Increment(x=w389) -> (x+1=w388:dbl)
                n194 = in-place-cluster #13("n false alarm"=w388) -> (w386:cluster{})
              }
              n195 = Bundle By Name(cluster=w386, "reward given"=TRUE) -> (w385:cluster{})
            }
          }
        }
        frame True {
          # "Reward subsystem has already finished for this trial"
        }
      }
    }
    frame Enabled {
    }
  }
